vi "tcsWEP_logEvent_sensorPssnList.vi"(8 "error in (no error)":errorcluster, 11 "logevent_sensorPssnList_Ctl":T1={"pssnList[31]"=[0.0, 0.0, 0.0, 0.0, 0.0, 0.0, 0.0, 0.0, 0.0, 0.0, 0.0, 0.0, 0.0, 0.0, 0.0, 0.0, 0.0, 0.0, 0.0, 0.0, 0.0, 0.0, 0.0, 0.0, 0.0, 0.0, 0.0, 0.0, 0.0, 0.0, 0.0], "sensorIdList[31]"=[0, 0, 0, 0, 0, 0, 0, 0, 0, 0, 0, 0, 0, 0, 0, 0, 0, 0, 0, 0, 0, 0, 0, 0, 0, 0, 0, 0, 0, 0, 0], "timestamp"=0.0, "priority"=0}) -> (0 "error out":errorcluster, 2 "function return":i32, 3 "logevent_sensorPssnList_Ctl out":T1)   [LabVIEW 2016, in "SALLV_tcsWEP.lvlib"]
doc: "int tcsWEP_shm_logEvent_sensorPssnListLV(tcsWEP_logevent_sensorPssnListLV *logevent_sensorPssnList_Ctl );"
uses:
  SALLV_tcsWEP.lvlib
  DataTypes/logevent_sensorPssnList.ctl
  SALLV_tcsWEP.so
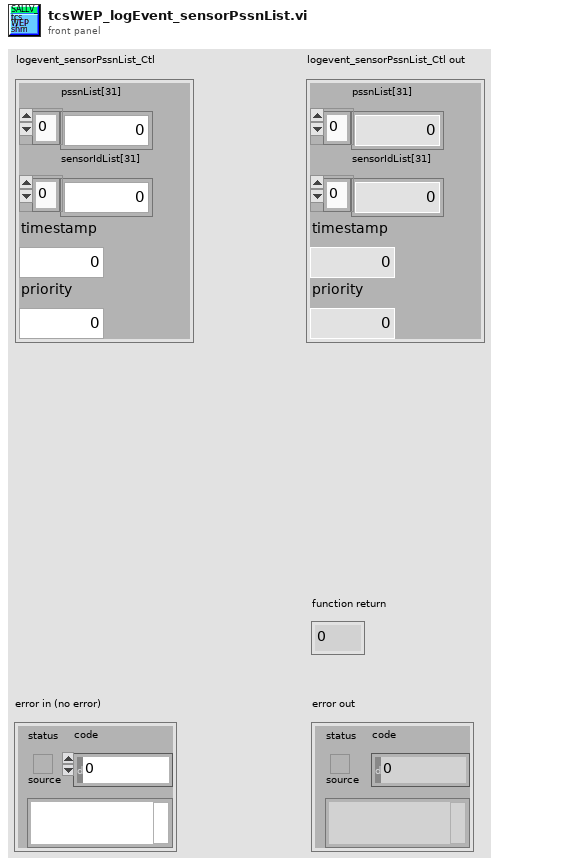
[diagram p1: front panel]
types:
  T1 = typedef "SALLV_tcsWEP.lvlib/logevent_sensorPssnList.ctl" = cluster{"pssnList[31]":dbl[], "sensorIdList[31]":i16[], "timestamp":dbl, "priority":i32}
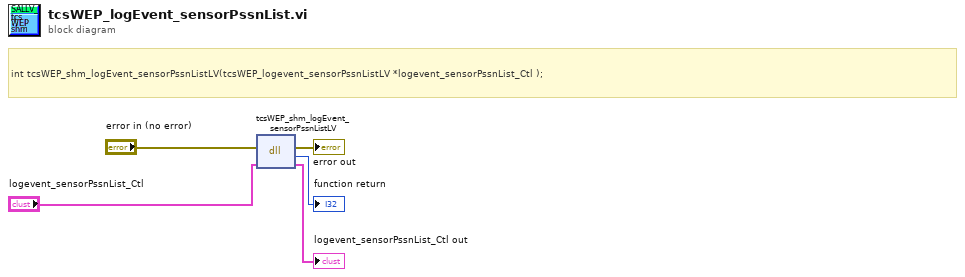
[diagram p0: block diagram]
diagram:
  # "int tcsWEP_shm_logEvent_sensorPssnListLV(tcsWEP_logevent_sensorPssnListLV *logevent_sensorPssnList_Ctl );"
  n1 = dll-call lib="home/ttsai/Documents/salAPI/SALLV_tcsWEP.*" fn="tcsWEP_shm_logEvent_sensorPssnListLV"(error in="error in (no error)", "logevent_sensorPssnList_Ctl"="logevent_sensorPssnList_Ctl") -> (error out=→"error out":errorcluster, →"function return":i32, "logevent_sensorPssnList_Ctl"=→"logevent_sensorPssnList_Ctl out":T1)  [unwired: 2 in, 1 out]
